vi "file.corrige caracteres prohibidos.vi"(1 "ASIC'S Number 2":string) -> (0 "ASIC'S Number":string)   [LabVIEW 2019]
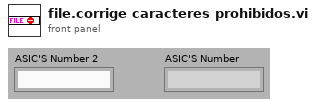
[diagram p1: front panel]
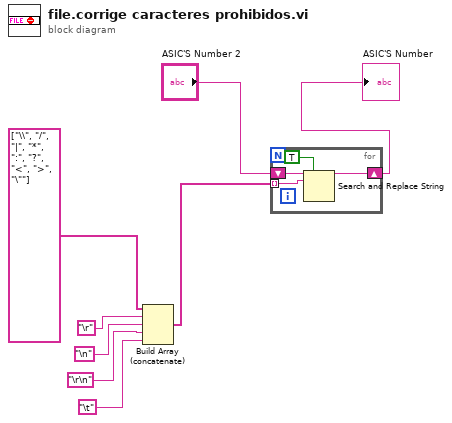
[diagram p0: block diagram]
diagram:
  n1 = Build Array (concatenate)(string[] ["\\", "/", "|", "*", ":", "?", "<", ">", "\""], "\r", "\n", "\r\n", "\t") -> (w5:string[])
  n2 = for {
    tunnel: w5 -> [w10] mode=indexing
    shift-right: [w9] -> w8
    shift-left: "ASIC'S Number 2" -> [w11]
    n3 = Search and Replace String(replace all?=TRUE ("replace all? (F)"), input string=w11, search string=w10) -> (result string=w9:string)  [unwired: 5 in, 3 out]
  }
  "ASIC'S Number" <- w8
